vi "Torque Props.vi"(8 "error in (no error)":errorcluster, 11 "Board Info for checking":T1) -> (0 "error out":errorcluster, 2 "scaling info out":variant, 3 "bridge info out":variant)   [LabVIEW 2010, in "PXIe-433x Custom Device.lvlib"]
uses:
  PXIe-433x Custom Device.lvlib
  Generic Bridge Information.ctl
  Torque Scaling Information.ctl
  Max Value.ctl
  Min Value.ctl
  Board Info for checking settings.ctl
  Scale Type.ctl
  Sensor Type.ctl
panel:
  in  "Minimum Value":T2=-5000.0 caption="lb-in"
  in  "Maximum Value":T3=5000.0 caption="lb-in"
  out "Error Description":string
  out "Tab Control":enum32{"No Error", "No Check", "Error"}(tab)
  out "Valid":bool=TRUE
  in  "No Error Check Details":bool
  out "No Check":bool=TRUE
  in  "Error Details":bool
  in  "stop":bool
  out "Valid Configuration?":bool
  in  "physical units":i32(ring)=15876 items=["Newtons"=15875, "Pounds"=15876, "kgf"=15877]
  in  "bridge information":T4={"bridge configuration"=10182, "voltage excitation source"=10200, "voltage excitation value"=2.5, "nominal bridge resistance"=350.0} {"voltage excitation source" items=["Internal"=10200, "External"=10167]; "bridge configuration" items=["Full Bridge"=10182, "Half Bridge"=10187, "Quarter Bridge"=10270]}
  in  "scaling information":T5={"first electrical value"=0.0, "second electrical value"=2.0, "electrical units"=15897, "first physical value"=0.0, "second physical value"=100.0, "physical units"=15883} {"physical units" items=["Nm"=15881, "oz-in"=15882, "lb-in"=15883, "lb-ft"=15884]; "electrical units" items=["Volts/Volt"=15896, "mVolts/Volt"=15897]}
  # "No Error"
  # "No Error"
  # "No Error Check"
  # "No Error Check"
  # "Error!"
  # "Error!"
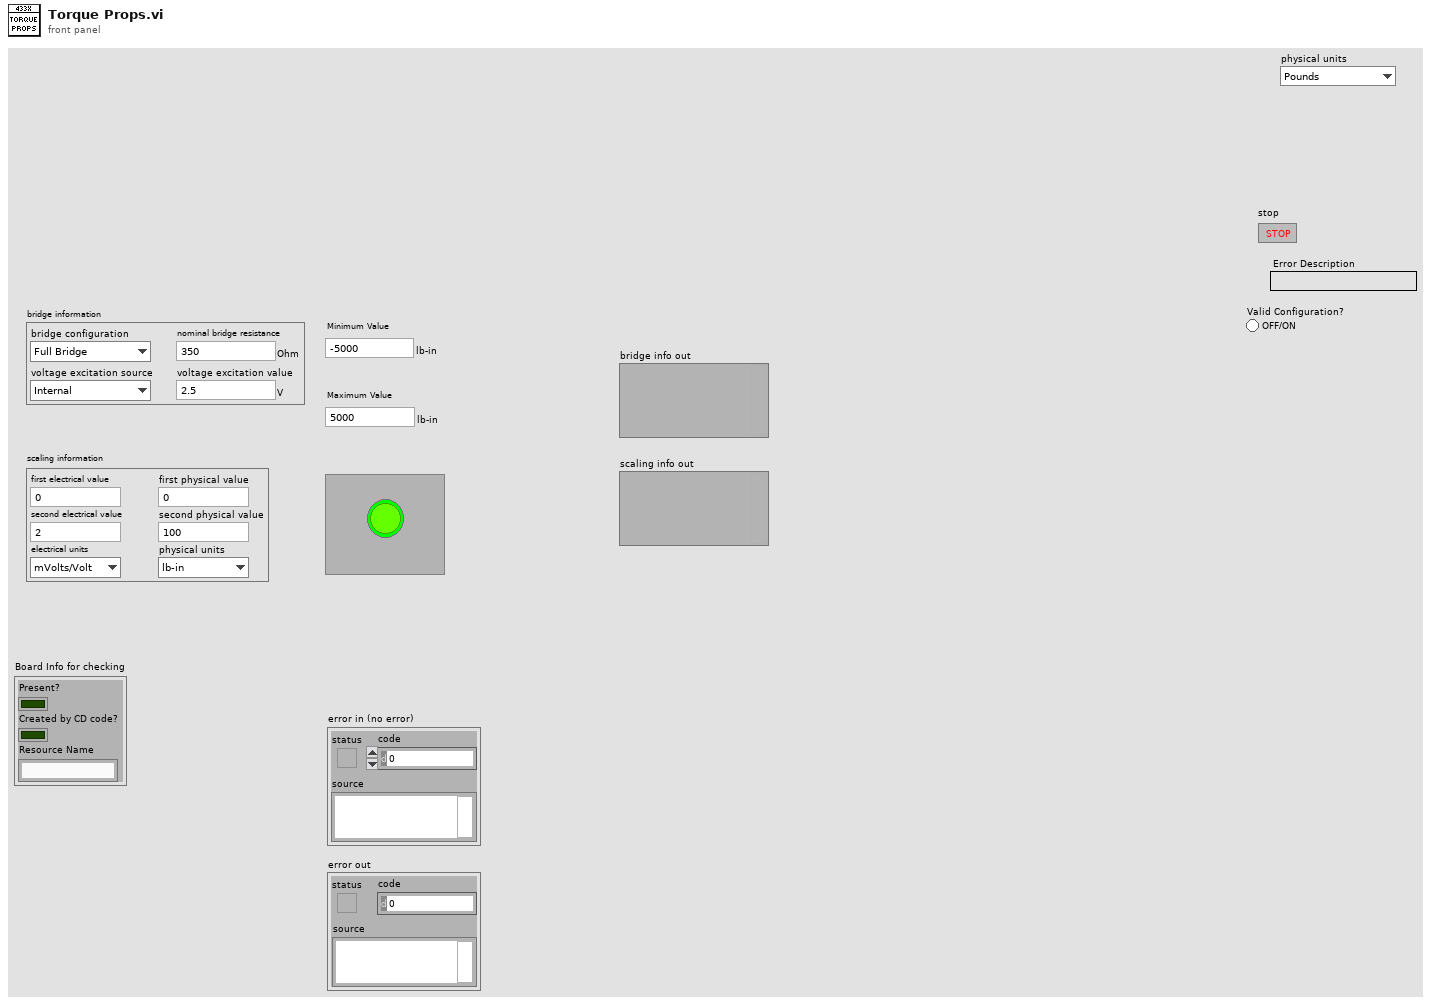
[diagram p1: front panel]
types:
  T1 = typedef "PXIe-433x Custom Device.lvlib/Board Info for checking settings.ctl" = cluster{"Present?":bool, "Created by CD code?":bool, "Resource Name":string}
  T2 = typedef "PXIe-433x Custom Device.lvlib/Min Value.ctl" = dbl
  T3 = typedef "PXIe-433x Custom Device.lvlib/Max Value.ctl" = dbl
  T4 = typedef "PXIe-433x Custom Device.lvlib/Generic Bridge Information.ctl" = cluster{"bridge configuration":i32, "voltage excitation source":i32, "voltage excitation value":dbl, "nominal bridge resistance":dbl}
  T5 = typedef "PXIe-433x Custom Device.lvlib/Torque Scaling Information.ctl" = cluster{"first electrical value":dbl, "second electrical value":dbl, "electrical units":i32, "first physical value":dbl, "second physical value":dbl, "physical units":i32}
  T6 = typedef "PXIe-433x Custom Device.lvlib/Scale Type.ctl" = enum16{"Linear", "Table", "Polynomial"}
  T7 = typedef "PXIe-433x Custom Device.lvlib/Sensor Type.ctl" = enum16{"Strain", "Force", "Pressure", "Torque"}
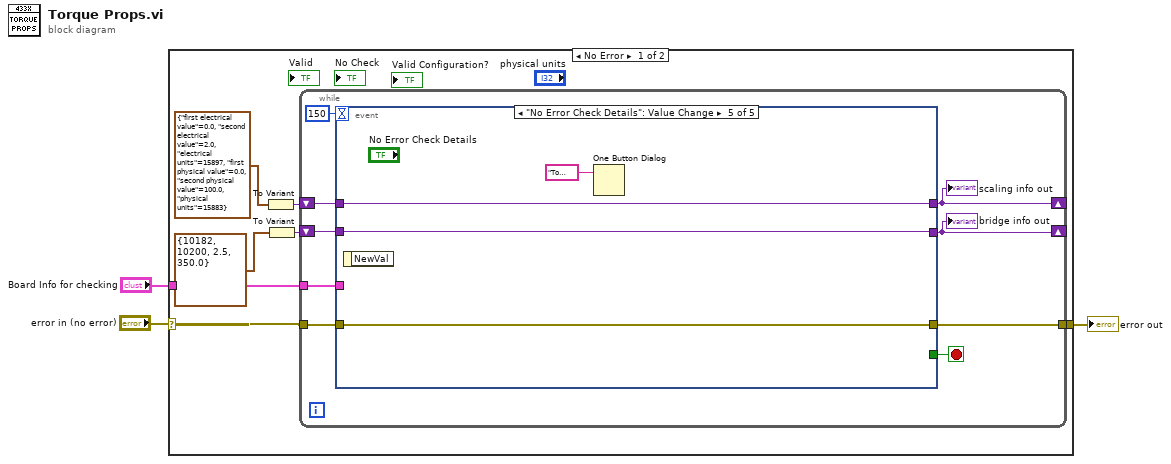
[diagram p0: block diagram]
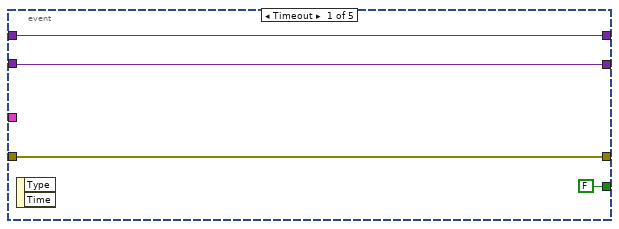
[diagram p2: hidden frame]
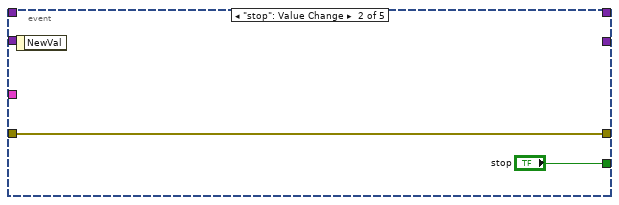
[diagram p3: hidden frame]
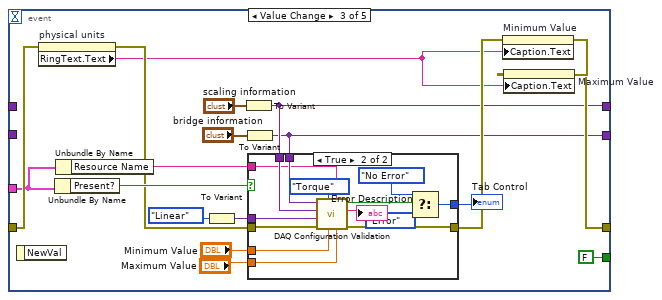
[diagram p4: hidden frame]
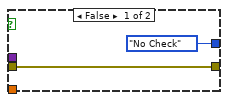
[diagram p5: hidden frame]
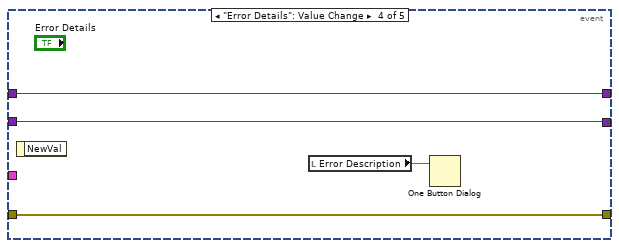
[diagram p6: hidden frame]
diagram:
  n1 = case shown="No Error" "error in (no error)" {
    selector: "error in (no error)" -> [w4 w69]
    tunnel: [w10 w69] -> w2
    tunnel: "Board Info for checking" -> [w5 _]
    frame No Error {
      n2 = To Variant(anything=T5 {"first electrical value"=0.0, "second electrical value"=2.0, "electrical units"=15897, "first physical value"=0.0, "second physical value"=100.0, "physical units"=15883} ("scaling information")) -> (Variant=w9:variant)
      n3 = To Variant(anything=T4 {"bridge configuration"=10182, "voltage excitation source"=10200, "voltage excitation value"=2.5, "nominal bridge resistance"=350.0} ("bridge information")) -> (Variant=w6:variant)
      n4 = while {
        tunnel: w4 -> [w19]
        tunnel: [w17] -> w10
        shift-right: [w15] -> _
        shift-left: w9 -> [w14]
        shift-right: [w13] -> _
        shift-left: w6 -> [w12]
        tunnel: w5 -> [w11]
        stop <- w18 stop-if-true
        n5 = event shown="[4] \"No Error Check Details\": Value Change" {
          selector: _ -> [_ _ _ _ _]
          dyn-events: _ -> [_ _ _ _ _]
          timeout: 150 -> [_ _ _ _ _]
          tunnel: w19 -> [w22 w24 w32 w64 w68]
          tunnel: [FALSE ("stop") "stop" FALSE ("stop") _ _] -> w18
          tunnel: [w22 w24 w35 w64 w68] -> w17
          tunnel: [w21 _ w29 w61 w66] -> w15
          tunnel: w14 -> [w21 _ _ w61 w66]
          tunnel: [w20 _ w28 w62 w67] -> w13
          tunnel: w12 -> [w20 _ _ w62 w67]
          tunnel: w11 -> [_ _ w27 _ _]
          event Timeout {
            n6 = event-data() -> ()  [unwired: 1 in, 2 out]
          }
          event "stop": Value Change {
            n7 = event-data() -> ()  [unwired: 1 in, 1 out]
          }
          event Value Change {
            n8 = event-data() -> ()  [unwired: 1 in, 1 out]
            n9 = property on="physical units" class="Ring (strict)"(error in=w32) -> (error out=w31:errorcluster, "RingText.Text"=w30:string)  [unwired: 1 in, 1 out]
            n10 = Unbundle By Name(w27) -> ("Present?"=w44:bool)
            n11 = Unbundle By Name(w27) -> ("Resource Name"=w26:string)
            n12 = To Variant(anything=Scale_Type."Linear" ("Scale Type")) -> (Variant=w39:variant)
            n13 = To Variant(anything="scaling information") -> (Variant=w29:variant)
            n14 = To Variant(anything="bridge information") -> (Variant=w28:variant)
            n15 = case shown="True" w44 {
              tunnel: w31 -> [w46 w60]
              tunnel: [w46 w53] -> w37
              tunnel: "Minimum Value" -> [_ w58]
              tunnel: "Maximum Value" -> [_ w57]
              tunnel: w29 -> [_ w55]
              tunnel: w28 -> [_ w56]
              tunnel: [enum32{"No Error", "No Check", "Error"}."No Check" ("Tab Control") w51] -> w40
              tunnel: w39 -> [_ w48]
              tunnel: w26 -> [_ w47]
              frame False {
              }
              frame True {
                n16 = call "DAQ Configuration Validation.vi"("Maximum Value"=w57, "DAQ Resource Name"=w47, "Minimum Value"=w58, "Sensor Type"=Sensor_Type."Torque", "error in"=w60, "scale type"=w48, "scaling info"=w55, "bridge info"=w56) -> ("error IO"=w53:errorcluster, "Error Source"=→"Error Description":string, "Valid configuration?"=w49:bool)  [unwired: 1 in]
                n17 = Select(t=enum32{"No Error", "No Check", "Error"}."No Error" ("Tab Control"), s=w49, f=enum32{"No Error", "No Check", "Error"}."Error" ("Tab Control")) -> (s? t:f=w51:enum32{"No Error", "No Check", "Error"})
              }
            }
            "Tab Control" <- w40
            n18 = property on="Minimum Value" class="DigNum (strict)"(error in=w37, "Caption.Text"=w30) -> (error out=w36:errorcluster)  [unwired: 1 in, 1 out]
            n19 = property on="Maximum Value" class="DigNum (strict)"(error in=w36, "Caption.Text"=w30) -> (error out=w35:errorcluster)  [unwired: 1 in, 1 out]
          }
          event "Error Details": Value Change {
            n20 = event-data() -> ()  [unwired: 1 in, 1 out]
            n21 = local read "Error Description"() -> (w63:string)
            n22 = One Button Dialog(message=w63) -> ()  [unwired: 1 in, 1 out]
          }
          event "No Error Check Details": Value Change {
            n23 = event-data() -> ()  [unwired: 1 in, 1 out]
            n24 = One Button Dialog(message="To perform error checking during Edition time, code needs either a physical local PXIe-433x or simulated one. One simulated couldn't be created, no error checking will be performed while editing settings. Error checking will still be performed while deploying Custom-Device.") -> ()  [unwired: 1 in, 1 out]
          }
        }
        "scaling info out" <- w15
        "bridge info out" <- w13
      }
    }
    frame Error {
    }
  }
  "error out" <- w2
